vi "秘钥转地址（btc.eth）.vi"(0 "私钥输入":string="a9ddf02d9a749a49db0c29eef84fdbcf82e7f3e3c63d1c989c2118296439e9da", 6 "error in (no error)":cluster{"状态":bool, "代码":i32, "源":string} caption="错误输入（无错误）") -> (20 "btc非压缩地址":string, 21 "btc压缩地址 2":string, 22 "eth地址":string, 26 "error out":cluster{"状态":bool, "代码":i32, "源":string} caption="错误输出")   [LabVIEW 2020]
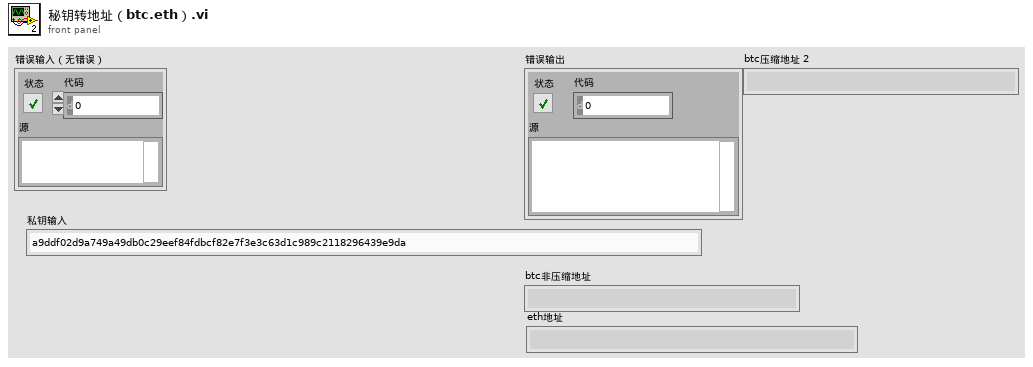
[diagram p1: front panel]
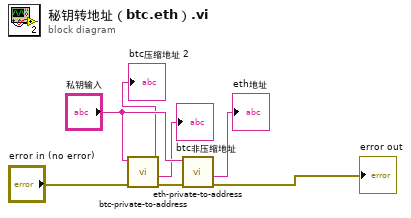
[diagram p0: block diagram]
diagram:
  n1 = call "btc-private-to-address.vi"("error in (no error)"="error in (no error)", "私钥输入"="私钥输入") -> ("error out"=w7:cluster{"状态":bool, "代码":i32, "源":string}, "非压缩地址"=→"btc非压缩地址":string, "压缩地址"=→"btc压缩地址 2":string)  [unwired: 7 in]
  n2 = call "eth-private-to-address.vi"("error in (no error)"=w7, "私钥输入"="私钥输入") -> ("error out"=→"error out":cluster{"状态":bool, "代码":i32, "源":string}, "地址"=→"eth地址":string)  [unwired: 8 in]
